vi "IC_Buffer_to_Picture.vi"(0 "Item":i32, 1 "ICImagingControl In":refnum<k7>, 2 "Error In (no error)":errorcluster) -> (3 "ICImagingControl Out":refnum<k7>, 4 "Picture Out":picture, 5 "SampleStartTime":dbl, 6 "Error Out":errorcluster)   [LabVIEW 2017]
uses:
  <vilib>/picture/picture.llb/Draw 8-Bit Pixmap.vi
  <vilib>/picture/picture.llb/Draw True-Color Pixmap.vi
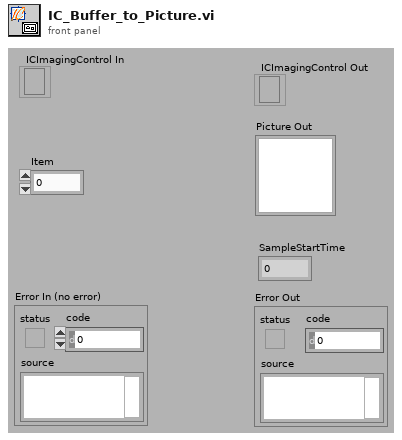
[diagram p1: front panel]
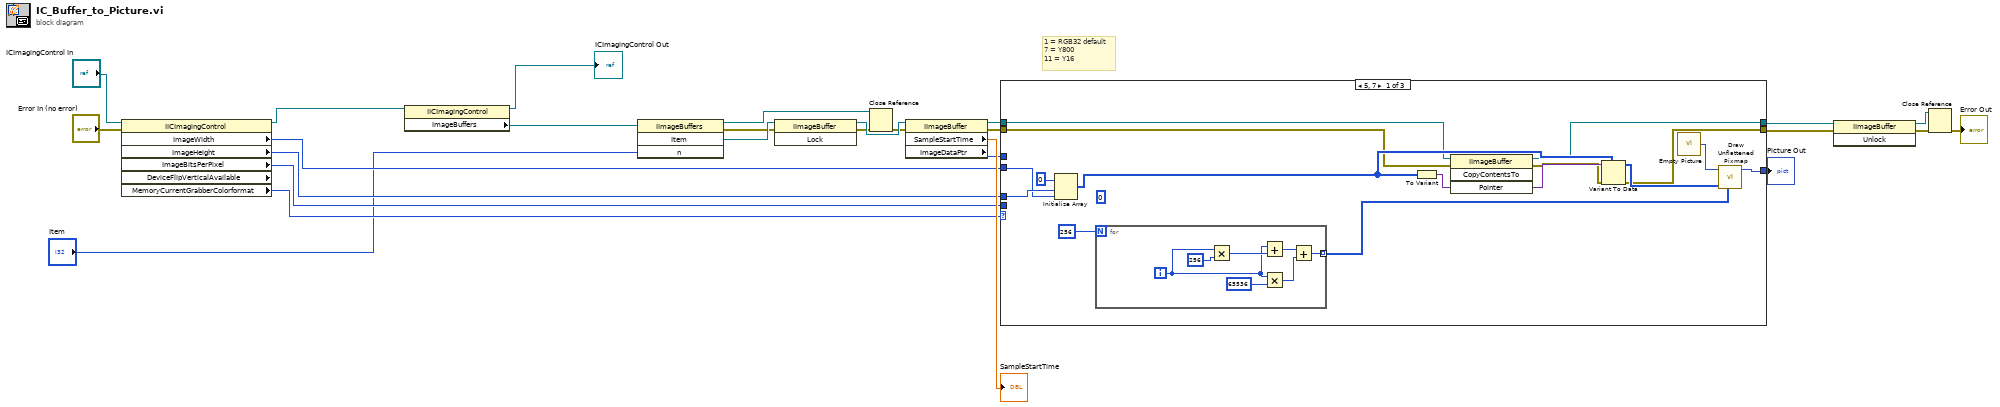
[diagram p0: block diagram]
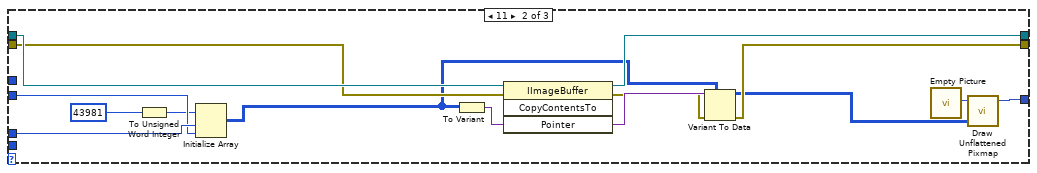
[diagram p2: hidden frame]
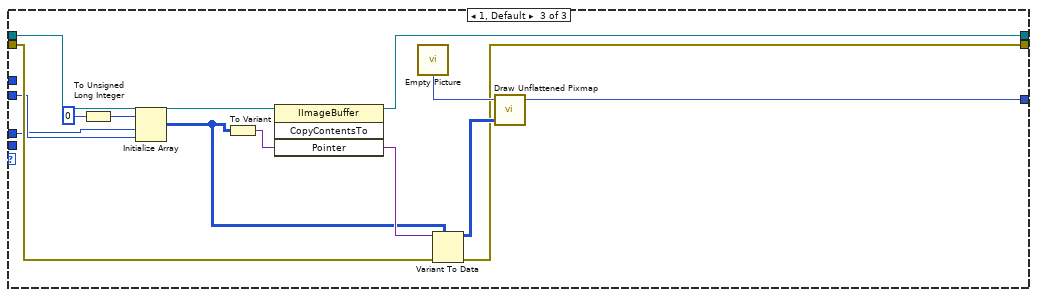
[diagram p3: hidden frame]
diagram:
  # "1 = RGB32 default\n7 = Y800\n11 = Y16"
  n1 = property class="IICImagingControl" props=["ImageWidth", "ImageHeight", "ImageBitsPerPixel", "DeviceFlipVerticalAvailable", "MemoryCurrentGrabberColorformat"](reference="ICImagingControl In", error in="Error In (no error)") -> (reference out=w3:refnum<k7>, "ImageWidth"=w12:i32, "ImageHeight"=w13:i32, "ImageBitsPerPixel"=w11:i32, "MemoryCurrentGrabberColorformat"=w14:i32)  [unwired: 2 out]
  n2 = property class="IICImagingControl"(reference=w3) -> (reference out=→"ICImagingControl Out":refnum<k7>, "ImageBuffers"=w1:refnum<k7>)  [unwired: 1 in, 1 out]
  n3 = invoke class="IImageBuffers" method="Item"(reference=w1, "n"="Item") -> (reference out=w23:refnum<k7>, error out=w18:errorcluster, "Item"=w19:refnum<k7>)  [unwired: 2 in, 1 out]
  n4 = invoke class="IImageBuffer" method="Lock"(reference=w19, error in=w18) -> (reference out=w17:refnum<k7>, error out=w16:errorcluster)  [unwired: 1 in, 1 out]
  n5 = Close Reference(reference=w23, error in (no error)=w16) -> (error out=w15:errorcluster)
  n6 = property class="IImageBuffer"(reference=w17, error in=w15) -> (reference out=w6:refnum<k7>, error out=w8:errorcluster, "SampleStartTime"=→"SampleStartTime":dbl, "ImageDataPtr"=w10:i64)
  n7 = case shown="5, 7" w14 {
    tunnel: w13 -> [w38 w63 w67]
    tunnel: w12 -> [w37 w62 w68]
    tunnel: w11 -> [_ _ _]
    tunnel: w10 -> [_ _ _]
    tunnel: [w36 w61 w75] -> w9
    tunnel: w8 -> [w31 w53 w70]
    tunnel: [w29 w52 w69] -> w7
    tunnel: w6 -> [w28 w55 w74]
    tunnel: [w27 w54 w73] -> w5
    frame 5, 7 {
      (unwired) 0
      n8 = Initialize Array(u8 0, w38, w37) -> (w33:u8[][])
      n9 = for {
        N: 256 -> [_]
        tunnel: [w43] -> w39 mode=indexing
        i -> [w44]
        n10 = Multiply(x=w44, y=256) -> (x*y=w47:i32)
        n11 = Add(x=w44, y=w47) -> (x+y=w45:i32)
        n12 = Multiply(x=w44, y=65536) -> (x*y=w49:i32)
        n13 = Add(x=w45, y=w49) -> (x+y=w43:i32)
      }
      n14 = To Variant(anything=w33) -> (Variant=w35:variant)
      n15 = invoke class="IImageBuffer" method="CopyContentsTo"(reference=w28, error in=w31, "Pointer"=w35) -> (reference out=w27:refnum<k7>, error out=w30:errorcluster, "Pointer"=w34:variant)  [unwired: 1 in, 1 out]
      n16 = Variant To Data(error in=w30, type=w33, Variant=w34) -> (data=w32:u8[][], error out=w29:errorcluster)
      n17 = call "Empty Picture"() -> ("empty picture"=w42:picture)
      n18 = call-poly <vilib>:"Draw Unflattened Pixmap.vi"("picture"=w42, "data"=w32, "color table"=w39) -> ("new picture"=w36:picture)  [unwired: 6 in]
    }
    frame 11 {
      n19 = To Unsigned Word Integer(number=u16 43981) -> (unsigned 16bit integer=w59:u16)
      n20 = Initialize Array(w59, w63, w62) -> (w51:u16[][])
      n21 = To Variant(anything=w51) -> (Variant=w58:variant)
      n22 = invoke class="IImageBuffer" method="CopyContentsTo"(reference=w55, error in=w53, "Pointer"=w58) -> (reference out=w54:refnum<k7>, error out=w56:errorcluster, "Pointer"=w57:variant)  [unwired: 1 in, 1 out]
      n23 = Variant To Data(error in=w56, type=w51, Variant=w57) -> (data=w50:u16[][], error out=w52:errorcluster)
      n24 = call "Empty Picture"() -> ("empty picture"=w64:picture)
      n25 = call-poly <vilib>:"Draw Unflattened Pixmap.vi"("picture"=w64, "data"=w50) -> ("new picture"=w61:picture)  [unwired: 7 in]
    }
    frame 1, Default {
      n26 = To Unsigned Long Integer(number=u8 0) -> (unsigned 32bit integer=w76:u32)
      n27 = Initialize Array(w76, w67, w68) -> (w66:u32[][])
      n28 = To Variant(anything=w66) -> (Variant=w65:variant)
      n29 = invoke class="IImageBuffer" method="CopyContentsTo"(reference=w74, "Pointer"=w65) -> (reference out=w73:refnum<k7>, "Pointer"=w72:variant)  [unwired: 2 in, 2 out]
      n30 = call "Empty Picture"() -> ("empty picture"=w78:picture)
      n31 = Variant To Data(error in=w70, type=w66, Variant=w72) -> (data=w71:u32[][], error out=w69:errorcluster)
      n32 = call-poly <vilib>:"Draw Unflattened Pixmap.vi"("picture"=w78, "data (RGB format)"=w71) -> ("new picture"=w75:picture)  [unwired: 7 in]
    }
  }
  "Picture Out" <- w9
  n33 = invoke class="IImageBuffer" method="Unlock"(reference=w5, error in=w7) -> (reference out=w20:refnum<k7>, error out=w22:errorcluster)  [unwired: 1 in, 1 out]
  n34 = Close Reference(reference=w20, error in (no error)=w22) -> (error out=→"Error Out":errorcluster)
